vi "Get Class Images.vi"(8 "error in (no error)":errorcluster, 11 "Editor.lvclass in":refnum<data-value>) -> (0 "error out":errorcluster, 3 "Editor.lvclass out":refnum<data-value>)   [LabVIEW 2015, in "Editor.lvclass"]
uses:
  Editor.lvclass
  <vilib>/picture/picture.llb/imagedata.ctl
  Project.lvclass
  Step.lvclass
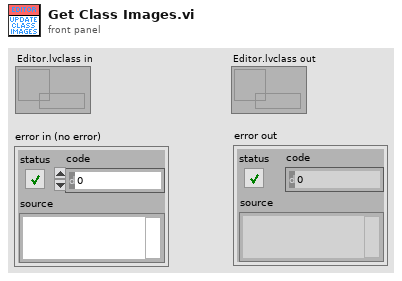
[diagram p1: front panel]
types:
  T1 = typedef "imagedata.ctl" = cluster{"image type":i32, "image depth":i32, "image":u8[], "mask":u8[], "colors":u32[], "Rectangle":cluster{"left":i16, "top":i16, "right":i16, "bottom":i16}}
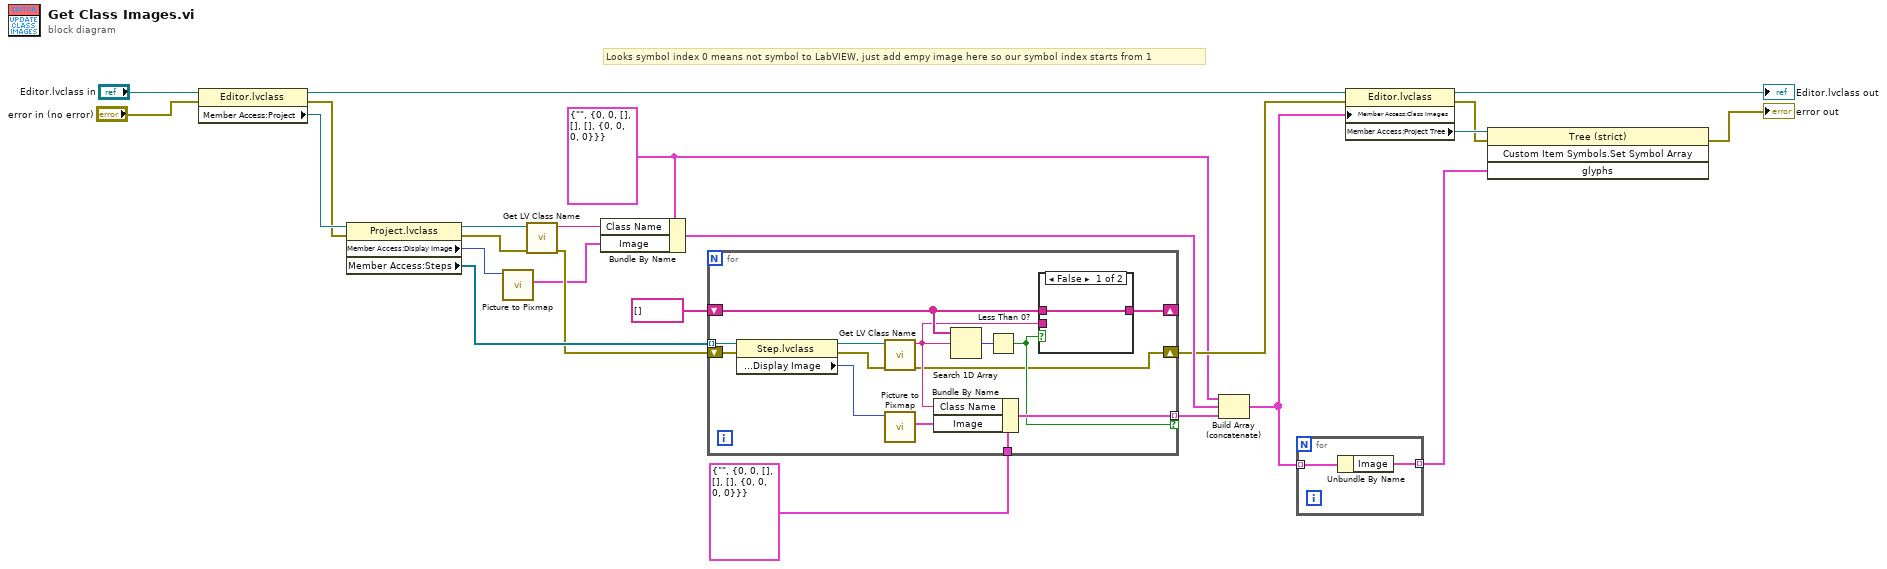
[diagram p0: block diagram]
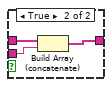
[diagram p2: hidden frame]
diagram:
  w1 = cluster{"Class Name":string, "Image":T1} {"Class Name"="", "Image"={"image type"=0, "image depth"=0, "image"=[], "mask"=[], "colors"=[], "Rectangle"={"left"=0, "top"=0, "right"=0, "bottom"=0}}}
  # "Looks symbol index 0 means not symbol to LabVIEW, just add empy image here so our symbol index starts from 1"
  n1 = property class="Editor.lvclass"(reference="Editor.lvclass in", error in="error in (no error)") -> (reference out=w5:refnum<data-value>, error out=w12:errorcluster, "Member Access:Project"=w14:refnum<class "Project.lvclass">)
  n2 = property class="Project.lvclass"(reference=w14, error in=w12) -> (reference out=w23:refnum<class "Project.lvclass">, error out=w24:errorcluster, "Member Access:Display Image"=w3:picture, "Member Access:Steps"=w21:refnum<class "Step.lvclass">[])
  n3 = call <vilib>:"Picture to Pixmap.vi"("picture"=w3) -> ("image data"=w2:T1)  [unwired: 9 in, 1 out]
  n4 = call <vilib>:"Get LV Class Name.vi"("error in (no error)"=w24, "object"=w23) -> ("error out"=w20:errorcluster, "class name"=w22:string)  [unwired: 8 in]
  n5 = Bundle By Name(cluster=w1, "Class Name"=w22, "Image"=w2) -> (w17:cluster{"Class Name":string, "Image":T1})
  n6 = for {
    tunnel: w21 -> [w38] mode=indexing
    shift-right: [w32] -> _
    shift-left: string[] [] -> [w33]
    tunnel: cluster{"Class Name":string, "Image":T1} {"Class Name"="", "Image"={"image type"=0, "image depth"=0, "image"=[], "mask"=[], "colors"=[], "Rectangle"={"left"=0, "top"=0, "right"=0, "bottom"=0}}} -> [w31]
    tunnel: [w29] -> w16 mode=indexing if=w28
    shift-right: [w27] -> w10
    shift-left: w20 -> [w36]
    n7 = property class="Step.lvclass"(reference=w38, error in=w36) -> (reference out=w37:refnum<class "Step.lvclass">, error out=w35:errorcluster, "Member Access:Display Image"=w26:picture)
    n8 = call <vilib>:"Get LV Class Name.vi"("error in (no error)"=w35, "object"=w37) -> ("error out"=w27:errorcluster, "class name"=w30:string)  [unwired: 8 in]
    n9 = call <vilib>:"Picture to Pixmap.vi"("picture"=w26) -> ("image data"=w25:T1)  [unwired: 9 in, 1 out]
    n10 = Bundle By Name(cluster=w31, "Class Name"=w30, "Image"=w25) -> (w29:cluster{"Class Name":string, "Image":T1})
    n11 = Search 1D Array(1D array=w33, element=w30) -> (index of element=w34:i32)  [unwired: 1 in]
    n12 = Less Than 0?(x=w34) -> (x < 0?=w28:bool)
    n13 = case shown="False" w28 {
      tunnel: w33 -> [w39 w42]
      tunnel: w30 -> [_ w41]
      tunnel: [w39 w40] -> w32
      frame False {
      }
      frame True {
        n14 = Build Array (concatenate)(w42, w41) -> (w40:string[])
      }
    }
  }
  n15 = Build Array (concatenate)(w1, w17, w16) -> (w11:cluster{"Class Name":string, "Image":T1}[])
  n16 = for {
    tunnel: w11 -> [w44] mode=indexing
    tunnel: [w43] -> w6 mode=indexing
    n17 = Unbundle By Name(w44) -> ("Image"=w43:T1)
  }
  n18 = property class="Editor.lvclass"(reference=w5, error in=w10, "Member Access:Class Images"=w11) -> (reference out=→"Editor.lvclass out":refnum<data-value>, error out=w8:errorcluster, "Member Access:Project Tree"=w9:refnum<vi>)
  n19 = invoke class="Tree (strict)" method="Custom Item Symbols.Set Symbol Array"(reference=w9, error in=w8, "glyphs"=w6) -> (error out=→"error out":errorcluster)  [unwired: 1 in, 3 out]
